vi "Cryostation.GET ALL.vi"(8 "error in (no error)":errorcluster, 11 "instrument.Cryostation in":refnum<class "instrument.Cryostation.lvclass">) -> (0 "error out":errorcluster, 2 "getAll":T1, 3 "instrument.Cryostation out":refnum<class "instrument.Cryostation.lvclass">)   [LabVIEW 2019, in "instrument.Cryostation.lvclass"]
uses:
  instrument.Cryostation.lvclass
  f9b1867d-c1be-4b22-ba65-52102b4d12d0.vi
  Typedefs/Cryostation.getAll--cluster.ctl
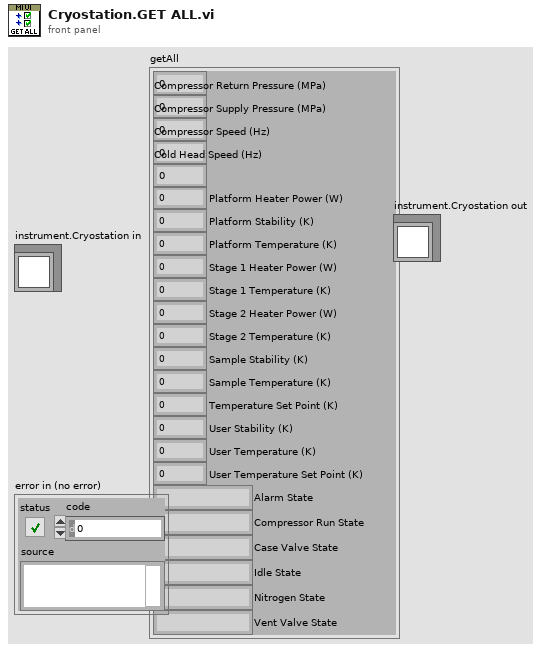
[diagram p1: front panel]
types:
  T1 = typedef "instrument.Cryostation.lvclass/Cryostation.getAll--cluster.ctl" = cluster{"Chamber Pressure (mTorr)":dbl, "Compressor Return Pressure (MPa)":dbl, "Compressor Supply Pressure (MPa)":dbl, "Compressor Speed (Hz)":dbl, "Cold Head Speed (Hz)":dbl, "Platform Heater Power (W)":dbl, "Platform Stability (K)":dbl, "Platform Temperature (K)":dbl, "Stage 1 Heater Power (W)":dbl, "Stage 1 Temperature (K)":dbl, "Stage 2 Heater Power (W)":dbl, "Stage 2 Temperature (K)":dbl, "Sample Stability (K)":dbl, "Sample Temperature (K)":dbl, "Temperature Set Point (K)":dbl, "User Stability (K)":dbl, "User Temperature (K)":dbl, "User Temperature Set Point (K)":dbl, "Alarm State":string, "Compressor Run State":string, "Case Valve State":string, "Idle State":string, "Nitrogen State":string, "Vent Valve State":string}
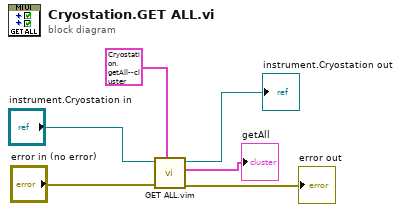
[diagram p0: block diagram]
diagram:
  n1 = call "GET ALL.vim"("type"=T1 {"Chamber Pressure (mTorr)"=0.0, "Compressor Return Pressure (MPa)"=0.0, "Compressor Supply Pressure (MPa)"=0.0, "Compressor Speed (Hz)"=0.0, "Cold Head Speed (Hz)"=0.0, "Platform Heater Power (W)"=0.0, "Platform Stability (K)"=0.0, "Platform Temperature (K)"=0.0, "Stage 1 Heater Power (W)"=0.0, "Stage 1 Temperature (K)"=0.0, "Stage 2 Heater Power (W)"=0.0, "Stage 2 Temperature (K)"=0.0, "Sample Stability (K)"=0.0, "Sample Temperature (K)"=0.0, "Temperature Set Point (K)"=0.0, "User Stability (K)"=0.0, "User Temperature (K)"=0.0, "User Temperature Set Point (K)"=0.0, "Alarm State"="", "Compressor Run State"="", "Case Valve State"="", "Idle State"="", "Nitrogen State"="", "Vent Valve State"=""} ("getAll"), "error in (no error)"="error in (no error)", "Instrument in"="instrument.Cryostation in") -> ("error out"=→"error out":errorcluster, "getAll"=→"getAll":T1, "Instrument out"=→"instrument.Cryostation out":refnum<class "instrument.Cryostation.lvclass">)  [unwired: 6 in]
